vi "AV Write.vi"   [LabVIEW 2023, in "Actual Value.lvclass"]
uses:
  Actual Value.lvclass
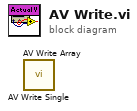
[diagram p0: block diagram]
diagram:
  n1 = call-dynamic "AV Write Single.vi"() -> ()  [unwired: 10 in, 2 out]
  n2 = call-dynamic "AV Write Array.vi"() -> ()  [unwired: 10 in, 2 out]
